vi "Utility_Find 1D Index of Selected array item.vi"(6 "Vertical(t)\nHorizontal(f)":bool, 7 "Border Size":i32=4, 8 "Error":errorcluster, 9 "Mouse Cord":T1, 11 "Array REf":refnum<vi>) -> (0 "Error Out":errorcluster, 1 "Valid Out":bool, 2 "Index Out":i32, 3 "Array REf Out":refnum<vi>)   [LabVIEW 2009]
doc: "Find Index of selected array item from mouse position"
uses:
  Controls/Cluster/Cluster_Mouse Location.ctl
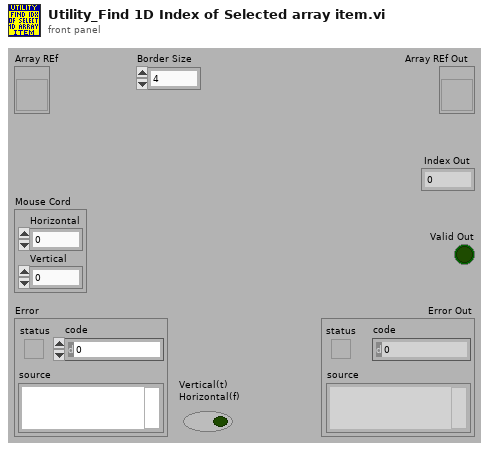
[diagram p1: front panel]
types:
  T1 = typedef "Cluster_Mouse Location.ctl" = cluster{"Horizontal":i32, "Vertical":i32}
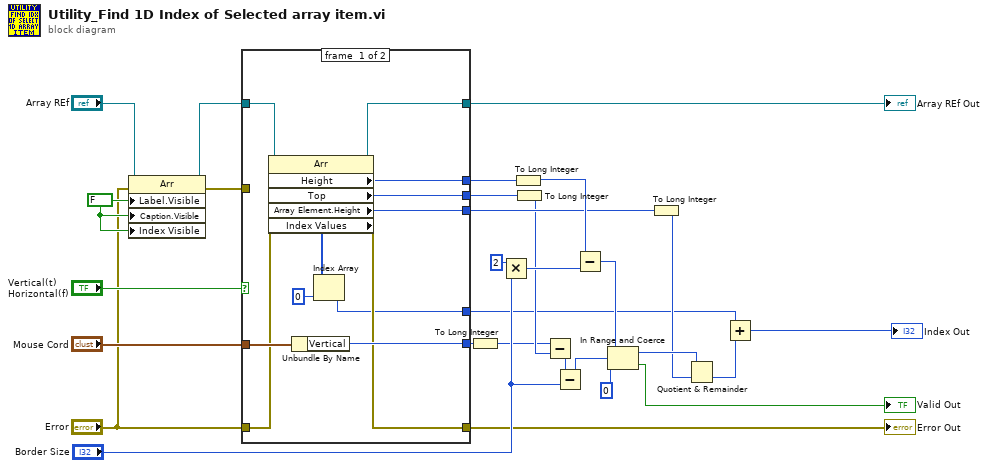
[diagram p0: block diagram]
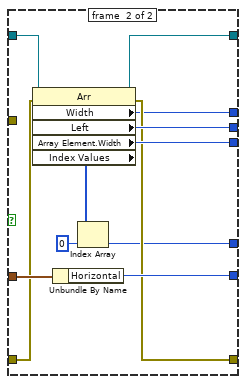
[diagram p2: hidden frame]
diagram:
  w17 = FALSE ("Label.Visible")
  n1 = property class="Arr"(reference="Array REf", error in="Error", "Label.Visible"=w17, "Caption.Visible"=w17, "Index Visible"=w17) -> (reference out=w18:refnum<vi>, error out=w6:errorcluster)
  n2 = case shown="True" "Vertical(t)\nHorizontal(f)" {
    tunnel: [w30 w42] -> w25
    tunnel: [w41 w53] -> w24
    tunnel: [w40 w52] -> w21
    tunnel: "Mouse Cord" -> [w39 w51]
    tunnel: w18 -> [w38 w50]
    tunnel: [w37 w49] -> w13
    tunnel: [w36 w48] -> w2
    tunnel: "Error" -> [w35 w47]
    tunnel: [w34 w46] -> w3
    tunnel: w6 -> [_ _]
    tunnel: [w31 w43] -> w5
    frame #0 {
      n3 = property class="Arr"(reference=w38, error in=w35) -> (reference out=w36:refnum<vi>, error out=w34:errorcluster, "Height"=w30:u32, "Top"=w41:i32, "Array Element.Height"=w37:u32, "Index Values"=w33:u32[])
      n4 = Unbundle By Name(w39) -> ("Vertical"=w40:i32)
      n5 = Index Array(array=w33, index=0) -> (element=w31:u32)
    }
    frame #1 {
      n6 = property class="Arr"(reference=w50, error in=w47) -> (reference out=w48:refnum<vi>, error out=w46:errorcluster, "Width"=w42:u32, "Left"=w53:i32, "Array Element.Width"=w49:u32, "Index Values"=w45:u32[])
      n7 = Unbundle By Name(w51) -> ("Horizontal"=w52:i32)
      n8 = Index Array(array=w45, index=0) -> (element=w43:u32)
    }
  }
  "Error Out" <- w3
  "Array REf Out" <- w2
  n9 = To Long Integer(number=w21) -> (32bit integer=w11:i32)
  n10 = Multiply(x=2, y="Border Size") -> (x*y=w16:i32)
  n11 = To Long Integer(number=w25) -> (32bit integer=w29:i32)
  n12 = To Long Integer(number=w24) -> (32bit integer=w12:i32)
  n13 = Subtract(x=w11, y=w12) -> (x-y=w22:i32)
  n14 = Subtract(x=w22, y="Border Size") -> (x-y=w23:i32)
  n15 = Subtract(x=w29, y=w16) -> (x-y=w26:i32)
  n16 = In Range and Coerce(upper limit=w26, x=w23, lower limit=0) -> (coerced(x)=w28:i32, In Range?=→"Valid Out":bool)
  n17 = To Long Integer(number=w13) -> (32bit integer=w10:i32)
  n18 = Quotient & Remainder(x=w28, y=w10) -> (floor(x/y)=w4:i32)  [unwired: 1 out]
  n19 = Add(x=w5, y=w4) -> (x+y=→"Index Out":u32)
